vi "Load and Split Signals.vi"(0 "Filename":path=path "E:/LabVIEW/Data/Test Data/Subj-Austin_Trial-1_Condition-None.lvm", 6 "Error In":errorcluster) -> (16 "Filename Out":path=path "E:/LabVIEW/Data/Test Data/Subj-Austin_Trial-1_Condition-None.lvm" caption="Filename", 17 "F0":dynamicdata(graph), 20 "Flow":dynamicdata(graph), 21 "EGG":dynamicdata(graph), 22 "SubGP":dynamicdata(graph), 23 "Audio":dynamicdata(graph), 24 "F0 (EGG)":dynamicdata(graph), 25 "SPL":dynamicdata(graph), 26 "Error Out":errorcluster, 27 "SupraGP":dynamicdata(graph))   [LabVIEW 2020, in "SubVIs.lvlib"]
uses:
  SubVIs.lvlib
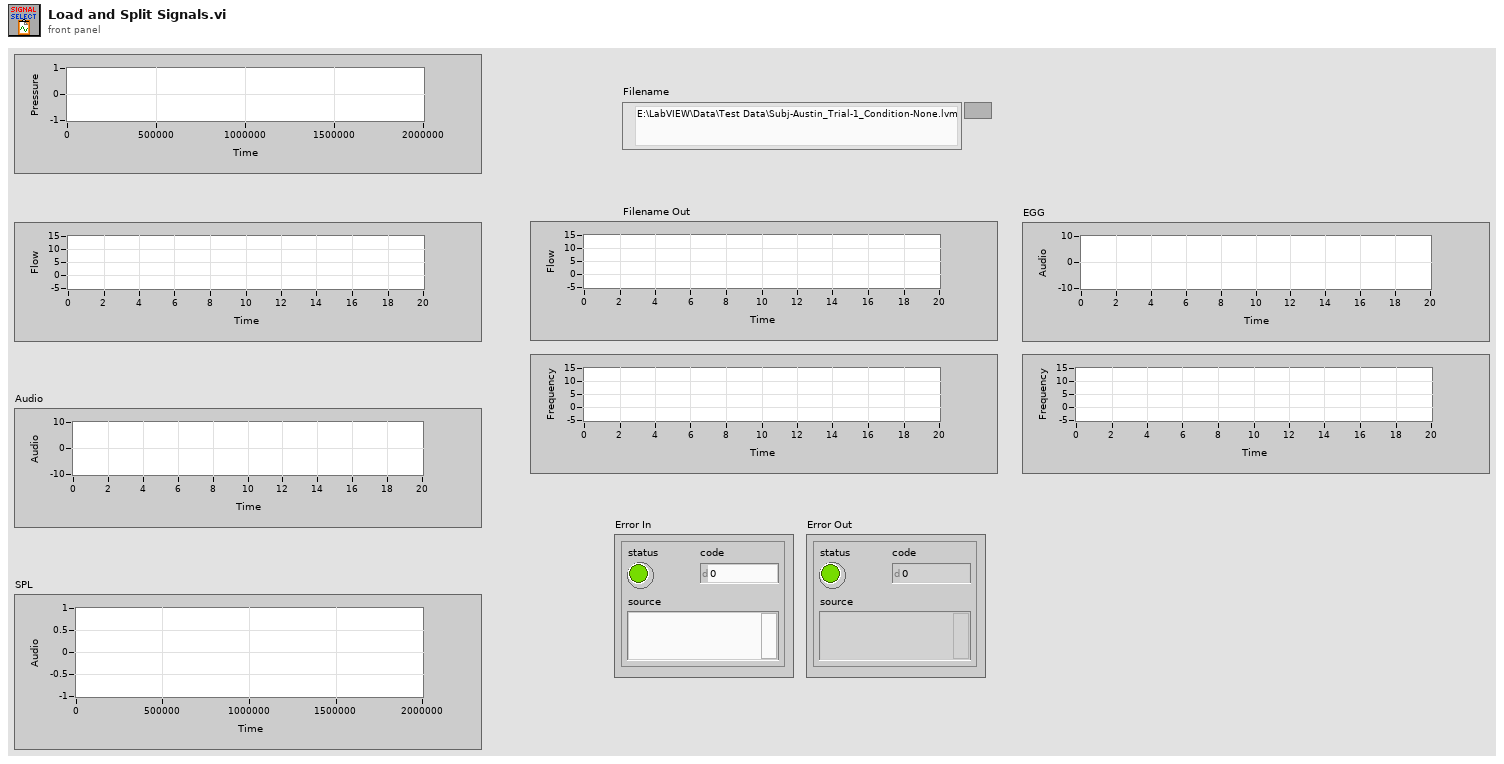
[diagram p1: front panel]
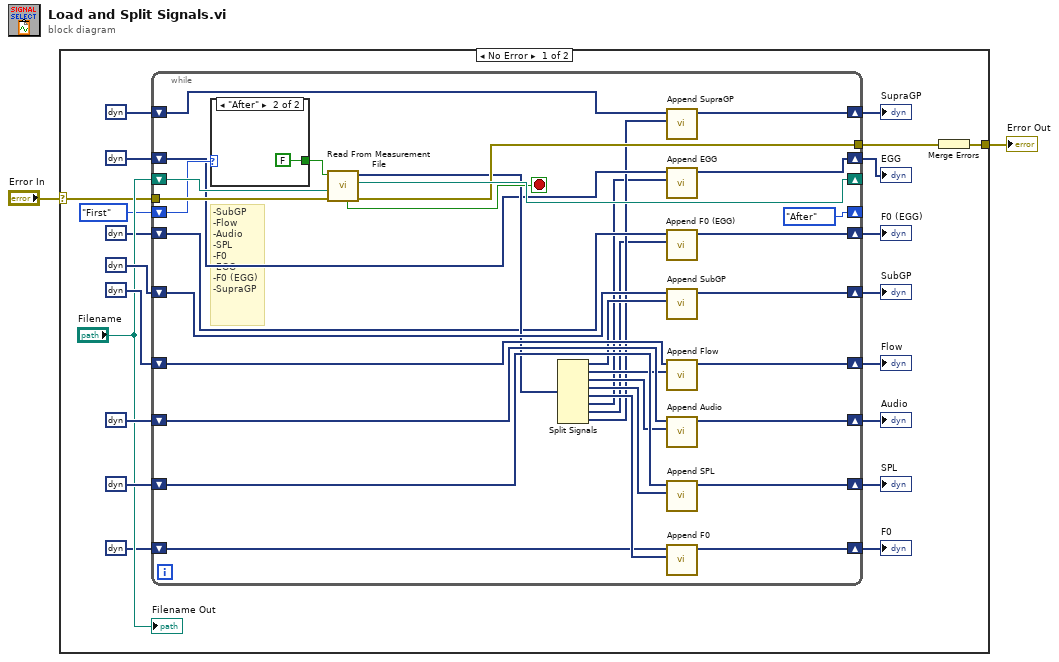
[diagram p0: block diagram]
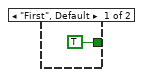
[diagram p2: hidden frame]
diagram:
  n1 = case shown="No Error" "Error In" {
    selector: "Error In" -> [w9 w59]
    tunnel: [w23 w59] -> w1
    frame No Error {
      n2 = while {
        shift-right: [w56] -> _
        shift-left: "Filename" -> [w53]
        shift-right: [w44] -> w17
        shift-left: dynamicdata [] ("Waveform Graph") -> [w51]
        shift-right: [w39] -> w13
        shift-left: dynamicdata [] ("Waveform Graph") -> [w50]
        shift-right: [w43] -> w16
        shift-left: dynamicdata [] ("Waveform Graph") -> [w49]
        shift-right: [w40] -> w15
        shift-left: dynamicdata [] ("Waveform Graph") -> [w48]
        shift-right: [enum16{"First", "After"}."After"] -> _
        shift-left: enum16{"First", "After"}."First" -> [w38]
        shift-right: [w33] -> w10
        shift-left: dynamicdata [] ("Waveform Graph") -> [w34]
        tunnel: w9 -> [w54]
        tunnel: [w55] -> w14
        shift-right: [w32] -> w5
        shift-left: dynamicdata [] ("Waveform Graph") -> [w28]
        shift-right: [w31] -> w4
        shift-left: dynamicdata [] ("Waveform Graph") -> [w27]
        shift-right: [w30] -> w3
        shift-left: dynamicdata [] ("Waveform Graph") -> [w29]
        stop <- w52 stop-if-true
        # "-SubGP\n-Flow\n-Audio\n-SPL\n-F0\n-EGG\n-F0 (EGG)\n-SupraGP"
        n3 = case shown="\"After\"" w38 {
          tunnel: [TRUE ("Reset") FALSE ("Reset")] -> w37
          frame "First", Default {
          }
          frame "After" {
          }
        }
        n4 = call "Read From Measurement File"("error in (no error)"=w54, "Filename"=w53, "Reset"=w37) -> ("error out"=w55:errorcluster, "Filename Out"=w56:path, "Signals"=w41:dynamicdata, "EOF?"=w52:bool)  [unwired: 3 in, 2 out]
        n5 = Split Signals(w41) -> (w47:dynamicdata, w46:dynamicdata, w45:dynamicdata, w42:dynamicdata, w35:dynamicdata, w25:dynamicdata, w24:dynamicdata, w26:dynamicdata)  [unwired: 8 in]
        n6 = call "Append SupraGP"("Input Signal B"=w26, "Input Signal A"=w28) -> ("Appended Signals"=w32:dynamicdata)  [unwired: 8 in, 1 out]
        n7 = call "Append EGG"("Input Signal B"=w25, "Input Signal A"=w27) -> ("Appended Signals"=w31:dynamicdata)  [unwired: 8 in, 1 out]
        n8 = call "Append F0 (EGG)"("Input Signal B"=w24, "Input Signal A"=w29) -> ("Appended Signals"=w30:dynamicdata)  [unwired: 8 in, 1 out]
        n9 = call "Append SubGP"("Input Signal B"=w47, "Input Signal A"=w51) -> ("Appended Signals"=w44:dynamicdata)  [unwired: 8 in, 1 out]
        n10 = call "Append Flow"("Input Signal B"=w46, "Input Signal A"=w50) -> ("Appended Signals"=w39:dynamicdata)  [unwired: 8 in, 1 out]
        n11 = call "Append Audio"("Input Signal B"=w45, "Input Signal A"=w49) -> ("Appended Signals"=w43:dynamicdata)  [unwired: 8 in, 1 out]
        n12 = call "Append SPL"("Input Signal B"=w42, "Input Signal A"=w48) -> ("Appended Signals"=w40:dynamicdata)  [unwired: 8 in, 1 out]
        n13 = call "Append F0"("Input Signal B"=w35, "Input Signal A"=w34) -> ("Appended Signals"=w33:dynamicdata)  [unwired: 8 in, 1 out]
      }
      "Flow" <- w13
      "SubGP" <- w17
      "SPL" <- w15
      "Audio" <- w16
      "F0" <- w10
      "SupraGP" <- w5
      "EGG" <- w4
      "F0 (EGG)" <- w3
      n14 = Merge Errors(w14) -> (w23:errorcluster)
      "Filename Out" <- "Filename"
    }
    frame Error {
    }
  }
  "Error Out" <- w1
